vi "Write Roles.vi"(8 "error in (no error)":errorcluster, 10 "Roles":T1, 11 "ZigZagPlay in":refnum<class "ZigZagPlay.lvclass">) -> (0 "error out":errorcluster, 3 "ZigZagPlay out":refnum<class "ZigZagPlay.lvclass">)   [LabVIEW 2020, in "ZigZagPlay.lvclass"]
uses:
  ZigZagPlay.lvclass
  ZigZagRole_class/ZigZagRole.lvclass
  ZigZagPlay.lvclass/ZigZagPlay.ctl
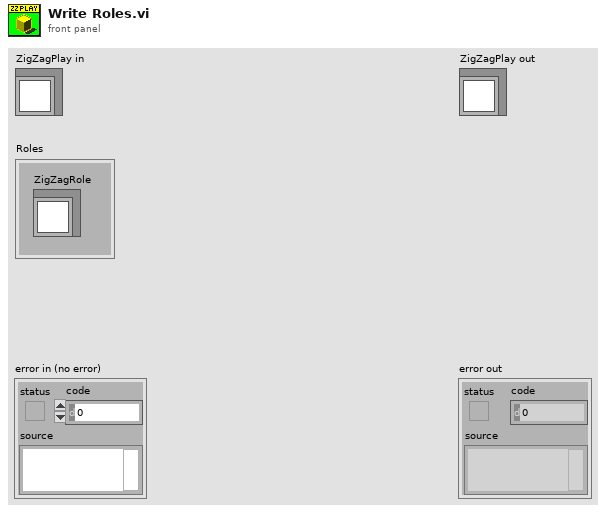
[diagram p1: front panel]
types:
  T1 = cluster{"ZigZagRole":refnum<class "ZigZagRole.lvclass">}
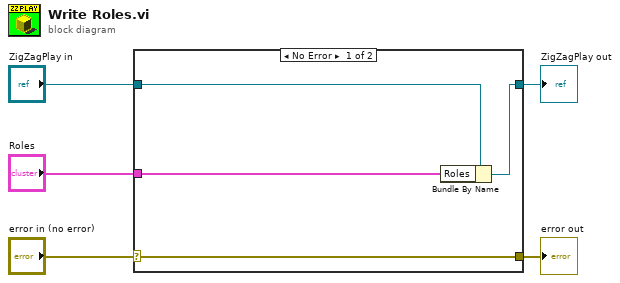
[diagram p0: block diagram]
diagram:
  n1 = case shown="No Error" "error in (no error)" {
    selector: "error in (no error)" -> [w9 w10]
    tunnel: [w9 w10] -> w4
    tunnel: [w7 w11] -> w2
    tunnel: "ZigZagPlay in" -> [w8 w11]
    tunnel: "Roles" -> [w6 _]
    frame No Error {
      n2 = Bundle By Name(cluster=w8, "Roles"=w6) -> (w7:refnum<class "ZigZagPlay.lvclass">)
    }
    frame Error {
    }
  }
  "error out" <- w4
  "ZigZagPlay out" <- w2
